vi "Main.vi"() -> ()   [LabVIEW 2018]
panel:
  out "Output":T1(array[cluster])
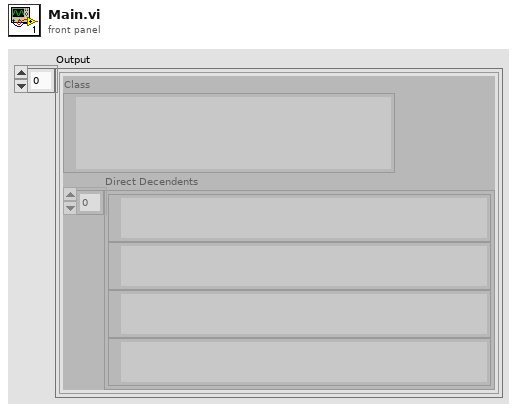
[diagram p1: front panel]
types:
  T1 = cluster{"Class":path, "Direct Decendents":path[]}[]
  T2 = cluster{"Class":path, "Direct Decendents":path[]}
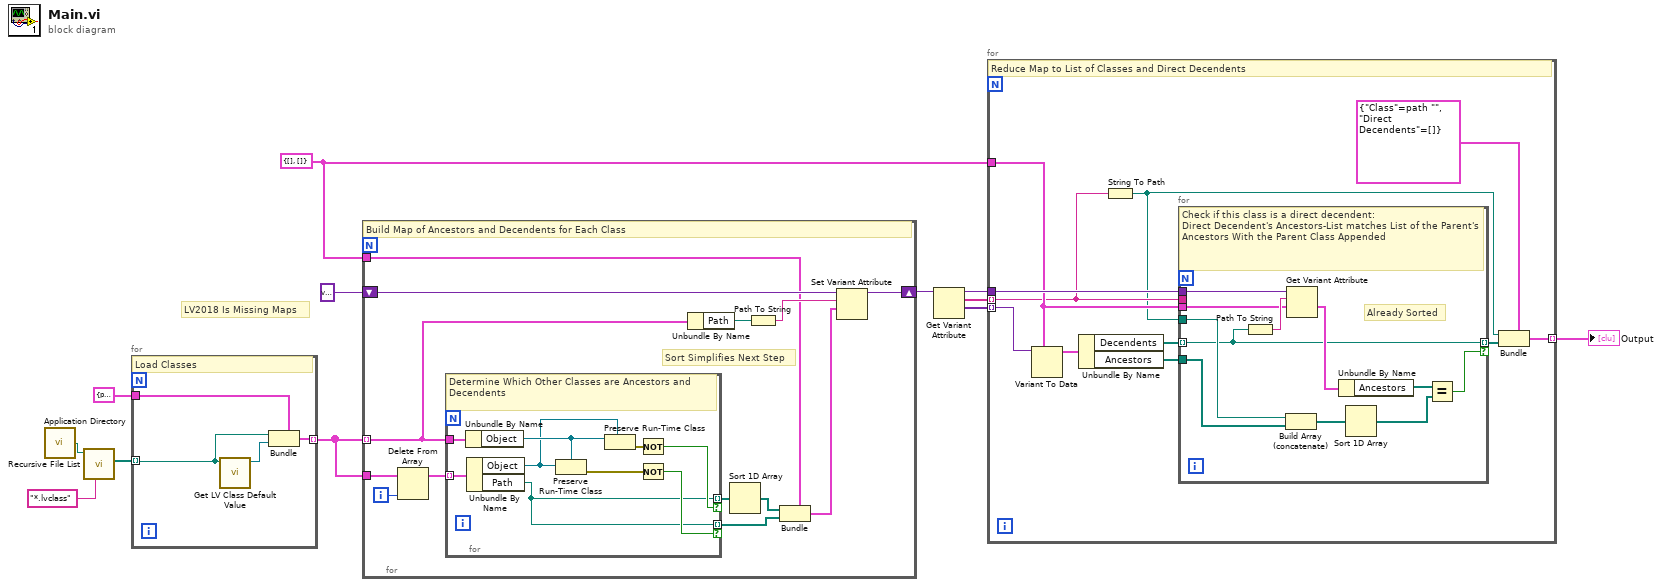
[diagram p0: block diagram]
diagram:
  w2 = cluster{"Ancestors":path[], "Decendents":path[]} {"Ancestors"=[], "Decendents"=[]} ("cluster")
  # "LV2018 Is Missing Maps"
  n1 = call <vilib>:"Application Directory.vi"() -> ("Application Directory"=w12:path)
  n2 = call <vilib>:"Recursive File List.vi"("pattern"="*.lvclass", "Folder Path"=w12) -> ("All Files in Dir"=w10:path[])  [unwired: 5 in, 4 out]
  n3 = for {
    tunnel: w10 -> [w16] mode=indexing
    tunnel: [w15] -> w9 mode=indexing
    tunnel: cluster{"Path":path, "Object":refnum<class>} {"Path"=path "", "Object"=refnum} ("cluster") -> [w14]
    # "Load Classes"
    n4 = call <vilib>:"Get LV Class Default Value.vi"("class path"=w16) -> ("object"=w13:refnum<class>)  [unwired: 9 in, 1 out]
    n5 = Bundle(cluster=w14, "Path"=w16, "Object"=w13) -> (w15:cluster{"Path":path, "Object":refnum<class>})
  }
  n6 = for {
    tunnel: w9 -> [w24] mode=indexing
    tunnel: w9 -> [w29]
    shift-right: [w25] -> w6
    shift-left: variant -> [w26]
    tunnel: w2 -> [w19]
    i -> [w28]
    # "Sort Simplifies Next Step"
    # "Build Map of Ancestors and Decendents for Each Class"
    n7 = Delete From Array(array=w29, index=w28) -> (array with subset deleted=w27:cluster{"Path":path, "Object":refnum<class>}[])  [unwired: 1 in, 1 out]
    n8 = for {
      tunnel: w27 -> [w33] mode=indexing
      tunnel: w24 -> [w36]
      tunnel: [w30] -> w17 mode=indexing if=w31
      tunnel: [w30] -> w20 mode=indexing if=w32
      # "Determine Which Other Classes are Ancestors and Decendents"
      n9 = Unbundle By Name(w36) -> ("Object"=w35:refnum<class>)
      n10 = Unbundle By Name(w33) -> ("Object"=w34:refnum<class>, "Path"=w30:path)
      n11 = Preserve Run-Time Class(object in=w34, 2:w35) -> (error out=w38:errorcluster)  [unwired: 1 in, 1 out]
      n12 = Preserve Run-Time Class(object in=w35, 2:w34) -> (error out=w37:errorcluster)  [unwired: 1 in, 1 out]
      n13 = Not(x=w37) -> (.not. x?=w32:bool)
      n14 = Not(x=w38) -> (.not. x?=w31:bool)
    }
    n15 = Unbundle By Name(w24) -> ("Path"=w23:path)
    n16 = Sort 1D Array(array=w20) -> (sorted array=w18:path[])
    n17 = Path To String(path=w23) -> (string=w22:string)
    n18 = Bundle(cluster=w19, "Ancestors"=w18, "Decendents"=w17) -> (w21:cluster{"Ancestors":path[], "Decendents":path[]})
    n19 = Set Variant Attribute(Variant=w26, name=w22, value=w21) -> (Variant out=w25:variant)  [unwired: 1 in, 2 out]
  }
  n20 = Get Variant Attribute(Variant=w6) -> (duplicate Variant=w4:variant, names=w5:string[], values=w3:variant[])  [unwired: 3 in, 1 out]
  n21 = for {
    tunnel: w5 -> [w43] mode=indexing
    tunnel: w4 -> [w48]
    tunnel: w3 -> [w47] mode=indexing
    tunnel: w2 -> [w46]
    tunnel: [w40] -> w1 mode=indexing
    # "Reduce Map to List of Classes and Direct Decendents"
    n22 = Variant To Data(type=w46, Variant=w47) -> (data=w45:cluster{"Ancestors":path[], "Decendents":path[]})  [unwired: 1 in, 1 out]
    n23 = Unbundle By Name(w45) -> ("Decendents"=w49:path[], "Ancestors"=w44:path[])
    n24 = String To Path(string=w43) -> (path=w41:path)
    n25 = for {
      tunnel: w49 -> [w51] mode=indexing
      tunnel: w48 -> [w60]
      tunnel: w46 -> [w58]
      tunnel: w43 -> [_]
      tunnel: w44 -> [w56]
      tunnel: w41 -> [w55]
      tunnel: [w51] -> w42 mode=indexing if=w50
      # "Already Sorted"
      # "Check if this class is a direct decendent:\nDirect Decendent's Ancestors-List matches List of the Parent's Ancestors With the Parent Class Appended"
      n26 = Path To String(path=w51) -> (string=w59:string)
      n27 = Build Array (concatenate)(w55, w56) -> (w54:path[])
      n28 = Get Variant Attribute(Variant=w60, name=w59, default value (empty Variant)=w58) -> (value=w57:cluster{"Ancestors":path[], "Decendents":path[]})  [unwired: 1 in, 3 out]
      n29 = Unbundle By Name(w57) -> ("Ancestors"=w53:path[])
      n30 = Sort 1D Array(array=w54) -> (sorted array=w52:path[])
      n31 = Equal?(x=w53, y=w52) -> (x = y?=w50:bool)
    }
    n32 = Bundle(cluster=T2 {"Class"=path "", "Direct Decendents"=[]}, "Class"=w41, "Direct Decendents"=w42) -> (w40:T2)
  }
  "Output" <- w1
